vi "Event handler-Ref plots.vi"(11 "Show ref plots window.NewVal":bool) -> ()   [LabVIEW 2017]
uses:
  Global Variables/General Globals.vi
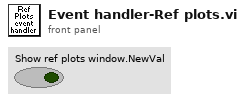
[diagram p1: front panel]
types:
  T1 = enum16{"Obtain queue", "Call window", "Call & send signal", "Release queue"}
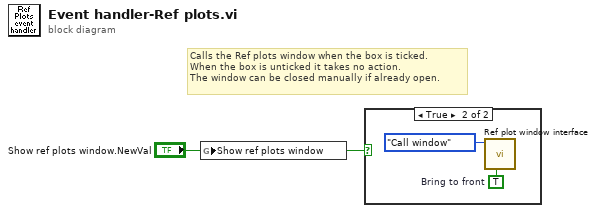
[diagram p0: block diagram]
diagram:
  # "Calls the Ref plots window when the box is ticked.\nWhen the box is unticked it takes no action.\nThe window can be closed manually if already open."
  n1 = global write "General Globals.vi" "Show ref plots window"("Show ref plots window.NewVal") -> ()
  n2 = case shown="True" "Show ref plots window.NewVal" {
    frame False {
    }
    frame True {
      w2 = TRUE  # Bring to front
      n3 = call "Ref plot window interface.vi"("Bring to front (F)"=w2, "Function"=T1."Call window") -> ()  [unwired: 8 in, 2 out]
    }
  }
